vi "DCON-ParseTempData.vi"(7 "Read Buffer":string) -> (8 "DataCluster":T1)   [LabVIEW 2019]
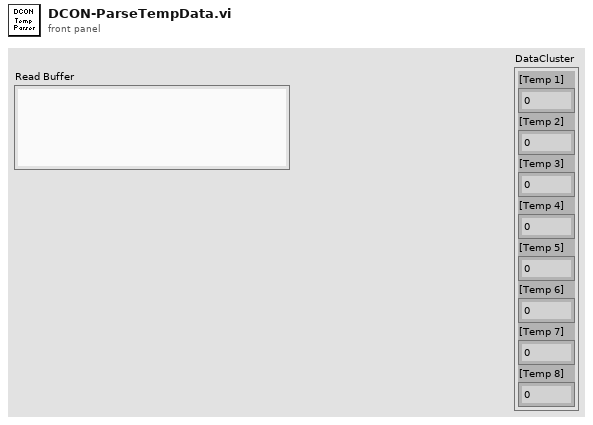
[diagram p1: front panel]
types:
  T1 = cluster{"[Temp 1]":dbl, "[Temp 2]":dbl, "[Temp 3]":dbl, "[Temp 4]":dbl, "[Temp 5]":dbl, "[Temp 6]":dbl, "[Temp 7]":dbl, "[Temp 8]":dbl}
  T2 = cluster{"Read Buffer":dbl, "Read Buffer":dbl, "Read Buffer":dbl, "Read Buffer":dbl, "Read Buffer":dbl, "Read Buffer":dbl, "Read Buffer":dbl, "Read Buffer":dbl}
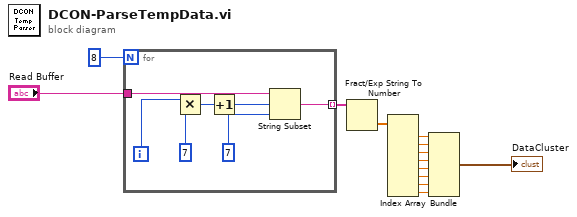
[diagram p0: block diagram]
diagram:
  n1 = for {
    N: 8 -> [_]
    tunnel: "Read Buffer" -> [w20]
    tunnel: [w15] -> w10 mode=indexing
    i -> [w19]
    n2 = Multiply(x=w19, y=7) -> (x*y=w17:i32)
    n3 = Increment(x=w17) -> (x+1=w14:i32)
    n4 = String Subset(string=w20, offset (0)=w14, length (rest)=7 ("length (rest)")) -> (substring=w15:string)
  }
  n5 = Fract/Exp String To Number(string=w10) -> (number=w9:dbl[])  [unwired: 3 in, 1 out]
  n6 = Index Array(array=w9) -> (element #1=w8:dbl, element #2=w7:dbl, element #3=w6:dbl, element #4=w5:dbl, element #5=w4:dbl, element #6=w3:dbl, element #7=w2:dbl, element #8=w1:dbl)  [unwired: 8 in]
  n7 = Bundle("Read Buffer"=w8, "Read Buffer"=w7, "Read Buffer"=w6, "Read Buffer"=w5, "Read Buffer"=w4, "Read Buffer"=w3, "Read Buffer"=w2, "Read Buffer"=w1) -> (→"DataCluster":T2)  [unwired: 1 in]
